vi "Create Enum Commands.vi"(8 "Enum Values":i32[](array[numeric]), 10 "Multi-line Text":string="\n", 11 "Commands":string) -> (3 "Result":string)   [LabVIEW 2018, in "Agilent MXA Series.lvlib"]
doc: "You can use this vi to create a command based on the input string, multi-line text and enum array."
uses:
  Agilent MXA Series.lvlib
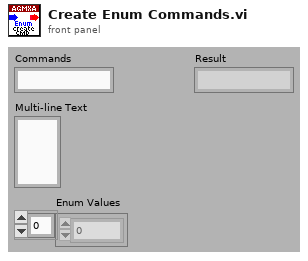
[diagram p1: front panel]
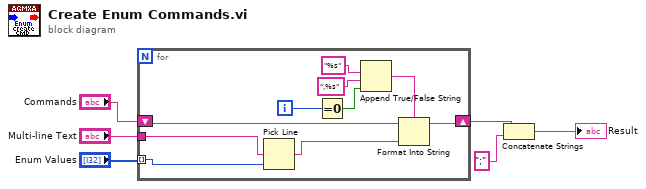
[diagram p0: block diagram]
diagram:
  n1 = for {
    tunnel: "Enum Values" -> [w9] mode=indexing
    shift-right: [w10] -> w5
    shift-left: "Commands" -> [w11]
    tunnel: "Multi-line Text" -> [w7]
    i -> [w12]
    n2 = Pick Line(multi-line string=w7, line index=w9) -> (output string=w8:string)  [unwired: 1 in]
    n3 = Equal To 0?(x=w12) -> (x = 0?=w13:bool)
    n4 = Append True/False String(1:w13, 2:",%s" ("format string"), 3:"%s" ("format string")) -> (0:w16:string)  [unwired: 1 in]
    n5 = Format Into String(format string=w16, initial string=w11, w8) -> (resulting string=w10:string)  [unwired: 1 in, 1 out]
  }
  n6 = Concatenate Strings(w5, ";" ("string")) -> (→"Result":string)
